vi "Ramp Pattern by Delta.vi"(9 "start":dbl, 10 "end":dbl=1.0, 11 "delta":dbl) -> (0 "error":i32, 2 "samples":i32, 3 "Ramp Pattern":dbl[](array[numeric]))   [LabVIEW 2011, in "NI_AALBase.lvlib"]
doc: "Generates an array containing a ramp pattern. You must manually select the polymorphic instance you want to use."
uses:
  NI_AALBase.lvlib
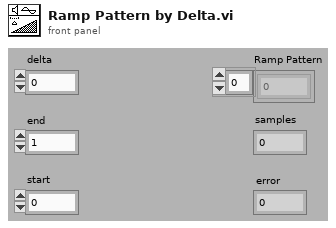
[diagram p1: front panel]
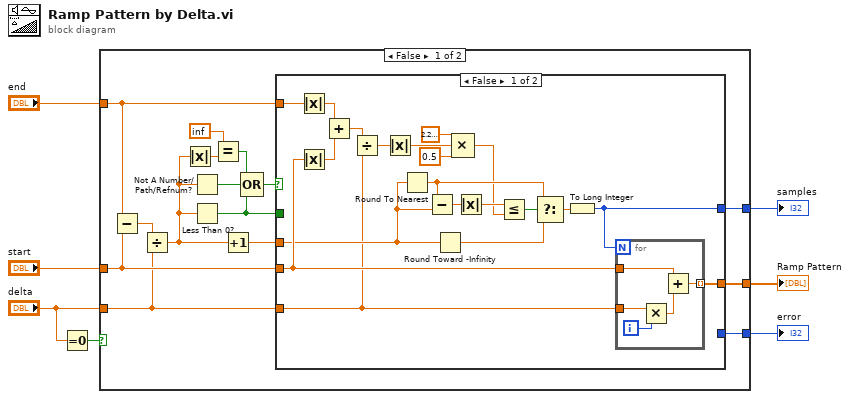
[diagram p0: block diagram]
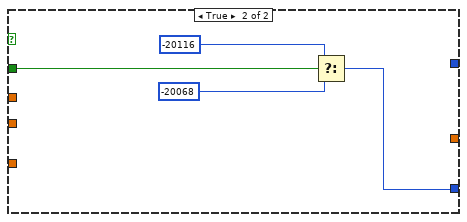
[diagram p2: hidden frame]
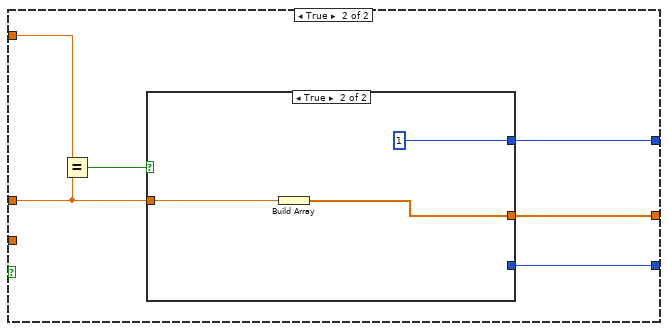
[diagram p3: hidden frame]
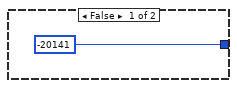
[diagram p4: hidden frame]
diagram:
  n1 = Equal To 0?(x="delta") -> (x = 0?=w2:bool)
  n2 = case shown="False" w2 {
    tunnel: "end" -> [w10 w56]
    tunnel: "start" -> [w21 w54]
    tunnel: [w20 w53] -> w5
    tunnel: [w19 w52] -> w4
    tunnel: "delta" -> [w18 _]
    tunnel: [w12 w57] -> w1
    frame False {
      n3 = Subtract(x=w10, y=w21) -> (x-y=w22:dbl)
      n4 = Divide(x=w22, y=w18) -> (x/y=w9:dbl)
      n5 = Absolute Value(x=w9) -> (abs(x)=w16:dbl)
      n6 = Not A Number/Path/Refnum?(number/path/refnum=w9) -> (NaN/Path/Refnum?=w14:bool)
      n7 = Less Than 0?(x=w9) -> (x < 0?=w11:bool)
      n8 = Equal?(x=inf, y=w16) -> (x = y?=w15:bool)
      n9 = Increment(x=w9) -> (x+1=w8:dbl)
      n10 = Compound Arithmetic op=OR(w15, w14, w11) -> (w13:bool)
      n11 = case shown="False" w13 {
        tunnel: w21 -> [w36 _]
        tunnel: [w42 _] -> w20
        tunnel: [w38 _] -> w19
        tunnel: w18 -> [w31 _]
        tunnel: [_ w49] -> w12
        tunnel: w11 -> [_ w51]
        tunnel: w10 -> [w37 _]
        tunnel: w8 -> [w33 _]
        frame False {
          n12 = Absolute Value(x=w37) -> (abs(x)=w35:dbl)
          n13 = Absolute Value(x=w36) -> (abs(x)=w34:dbl)
          n14 = Add(x=w35, y=w34) -> (x+y=w32:dbl)
          n15 = Divide(x=w32, y=w31) -> (x/y=w30:dbl)
          n16 = Absolute Value(x=w30) -> (abs(x)=w29:dbl)
          n17 = Round To Nearest(number=w33) -> (nearest integer value=w40:dbl)
          n18 = Subtract(x=w40, y=w33) -> (x-y=w27:dbl)
          n19 = Round Toward -Infinity(1:w33) -> (0:w41:dbl)
          n20 = Compound Arithmetic op=MULTIPLY(2.220446049250313e-16, w29, 0.5) -> (w25:dbl)
          n21 = Absolute Value(x=w27) -> (abs(x)=w26:dbl)
          n22 = Less Or Equal?(x=w26, y=w25) -> (x <= y?=w24:bool)
          n23 = Select(t=w40, s=w24, f=w41) -> (s? t:f=w39:dbl)
          n24 = To Long Integer(number=w39) -> (32bit integer=w38:i32)
          n25 = for {
            N: w38 -> [_]
            tunnel: w31 -> [w46]
            tunnel: w36 -> [w44]
            tunnel: [w43] -> w42 mode=indexing
            i -> [w47]
            n26 = Multiply(x=w46, y=w47) -> (x*y=w45:dbl)
            n27 = Add(x=w44, y=w45) -> (x+y=w43:dbl)
          }
        }
        frame True {
          n28 = Select(t=-20116, s=w51, f=-20068) -> (s? t:f=w49:i32)
        }
      }
    }
    frame True {
      n29 = Equal?(x=w56, y=w54) -> (x = y?=w55:bool)
      n30 = case shown="True" w55 {
        tunnel: [-20141 _] -> w57
        tunnel: w54 -> [_ w61]
        tunnel: [_ w60] -> w53
        tunnel: [_ 1] -> w52
        frame False {
        }
        frame True {
          n31 = Build Array(w61) -> (w60:dbl[])
        }
      }
    }
  }
  "error" <- w1
  "Ramp Pattern" <- w5
  "samples" <- w4
